vi "RunCalled.vi"(1 "TestResultMock In":refnum<class "TestResultMock.lvclass">) -> (0 "Run Called":bool)   [LabVIEW 2019, in "TestCaseTest.lvlib" / "Support.lvlib" / "TestResultMock.lvclass"]
uses:
  TestResultMock.lvclass
  TestResultMock.lvclass/TestResultMock.ctl
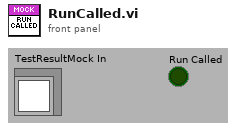
[diagram p1: front panel]
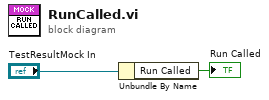
[diagram p0: block diagram]
diagram:
  n1 = Unbundle By Name("TestResultMock In") -> ("Run Called"=→"Run Called":bool)
